vi "Close_ Comm.vi"(8 "error in (no error)":errorcluster caption="entrée d'erreur (pas d'erreur)", 11 "Class Shielding_ Box en entrée":refnum<class "Class Shielding_ Box JC-PB3044.lvclass">) -> (0 "error out":errorcluster caption="sortie d'erreur", 3 "Class Shielding_ Box en sortie":refnum<class "Class Shielding_ Box JC-PB3044.lvclass">)   [LabVIEW 2020, in "Library Instrument & Equipement.lvlib" / "Library Shielding box.lvlib" / "Class Shielding_ Box JC-PB3044.lvclass"]
uses:
  Class Shielding_ Box JC-PB3044.lvclass
  C:/Users/ngarcin/OneDrive - Altyor/Standard TB/Class/Shielding box/Class Shielding box (Default)/Class Shielding_ Box (Default).lvclass
  Class Shielding_ Box JC-PB3044.lvclass/Class Shielding_ Box JC-PB3044.ctl
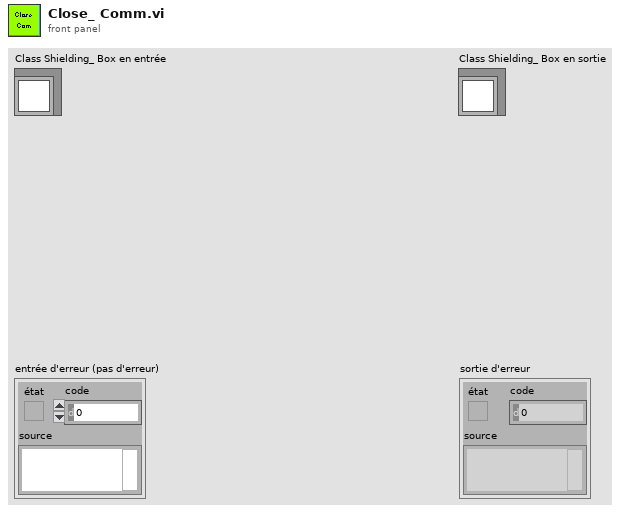
[diagram p1: front panel]
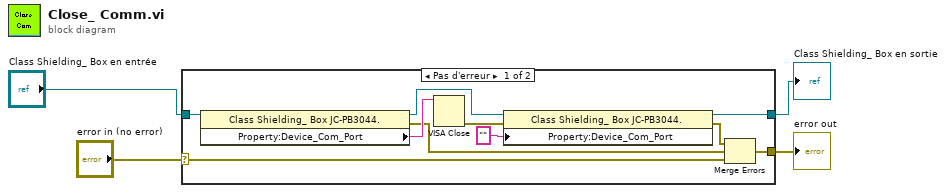
[diagram p0: block diagram]
diagram:
  n1 = case shown="Pas d'erreur" "error in (no error)" {
    selector: "error in (no error)" -> [w5 w16]
    tunnel: [w7 w16] -> w3
    tunnel: [w10 w15] -> w1
    tunnel: "Class Shielding_ Box en entrée" -> [w12 w15]
    frame No Error {
      n2 = property class="Class Shielding_ Box JC-PB3044."(reference=w12) -> (reference out=w11:refnum<class "Class Shielding_ Box JC-PB3044.lvclass">, error out=w6:errorcluster, "Property:Device_Com_Port"=w8:string)  [unwired: 1 in]
      n3 = VISA Close(VISA resource name=w8) -> (error out=w13:errorcluster)  [unwired: 1 in]
      n4 = property class="Class Shielding_ Box JC-PB3044."(reference=w11, error in=w13, "Property:Device_Com_Port"="" ("Address_Device")) -> (reference out=w10:refnum<class "Class Shielding_ Box JC-PB3044.lvclass">, error out=w9:errorcluster)
      n5 = Merge Errors(w9, w6, w5) -> (w7:errorcluster)
    }
    frame Error {
    }
  }
  "error out" <- w3
  "Class Shielding_ Box en sortie" <- w1
